vi "update.start_time.vi"(8 "error in (no error)":errorcluster, 10 "Start Time (now)":timestamp format="%<%x %.3X>T", 11 "Run in":refnum<class "Run.lvclass">) -> (0 "error out":errorcluster, 3 "Run out":refnum<class "Run.lvclass">)   [LabVIEW 2020, in "Run.lvclass"]
uses:
  Run.lvclass
  Run.lvclass/Run.ctl
  Nominal Client/Nominal Client.lvclass/Nominal Client.ctl
  Nominal Client/error.vi
  Nominal Client/trace.payload_sent.vi
  Nominal Client/trace.payload_received.vi
  Nominal Client/create.authorization_header.vi
  Nominal Client/error.vi/859f8e04-e495-489b-b5b4-7ac163f56130.vi
  Nominal Client/trace.calling_method.vi
  <vilib>/JDP Science/JDP Science Common Utilities/Trim Whitespace__JDP.vi
  <vilib>/AdvancedString/1D String Array to Delimited String.vi
  Nominal Client/api_token.get.vi
  <vilib>/Utility/libraryn.llb/Get File Extension.vi
  Nominal Client/log_file.write.vi
  <vilib>/JDP Science/JSONtext/Get all Object Items.vi
  <vilib>/Utility/error.llb/Error Cluster From Error Code.vi
  <vilib>/JDP Science/JSONtext/JSON text to Variant.vi
  <vilib>/JDP Science/JSONtext/LVClass Serializer/JSONtext LVClass Serializer.lvclass
  <vilib>/addons/_JKI.lib/REST Client/classes/Response Headers/Response Headers.lvclass
  <vilib>/addons/_JKI.lib/REST Client/classes/REST Client/REST Client.lvclass
  Nominal Client/Nominal Client.lvclass
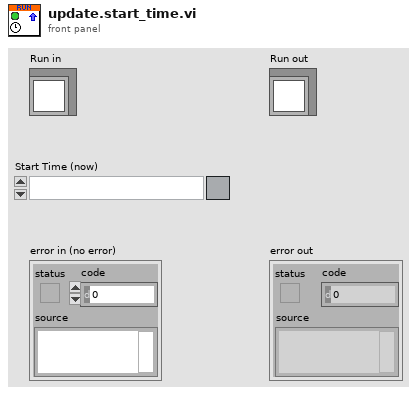
[diagram p1: front panel]
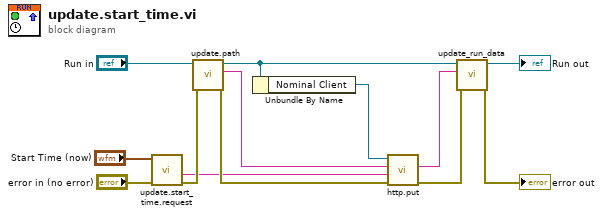
[diagram p0: block diagram]
diagram:
  n1 = call "update.start_time.request.vi"("error in"="error in (no error)", "start time"="Start Time (now)") -> ("error out"=w5:errorcluster, "Request"=w3:string)  [unwired: 8 in]
  n2 = call "update.path.vi"("error in"=w5, "Run"="Run in") -> ("error out"=w4:errorcluster, "path"=w12:string, "Run Out"=w10:refnum<class "Run.lvclass">)  [unwired: 7 in]
  n3 = Unbundle By Name(w10) -> ("Nominal Client"=w11:refnum<class "Nominal Client.lvclass">)
  n4 = call "http.put.vi"("error in"=w4, "Body"=w3, "Path"=w12, "Nominal Client in"=w11) -> ("error out"=w6:errorcluster, "Response"=w9:string)  [unwired: 4 in, 2 out]
  n5 = call "update_run_data.vi"("error in"=w6, "Run JSON"=w9, "Run in"=w10) -> ("error out"=→"error out":errorcluster, "Run out"=→"Run out":refnum<class "Run.lvclass">)  [unwired: 7 in]
